vi "Relay_Checker.vi"(0 "TSM context":T1) -> (15 "error out":errorcluster)   [LabVIEW 2019]
uses:
  <vilib>/NI_TestStand_SemiconductorModule/NI_TestStand_Semiconductor_Module.lvlibp/PinMap/General/SemiconductorModuleContext.ctl
  Common/Instrument Control/DCPower/TSM/TSM SSC DCPower.ctl
  <vilib>/NI_TestStand_SemiconductorModule/NI_TestStand_Semiconductor_Module.lvlibp/PinMap/PinQueryContext/MultiplePinMultipleSessionQueryContext/MultiplePinMultipleSessionQueryContext.lvclass
  Common/Instrument Control/DCPower/SSC DCPower/SSC DCPower.ctl
  Common/Instrument Control/Shared SubVIs/TSM Pin Abstraction/TSM Pin Information.ctl
  Common/Instrument Control/Shared SubVIs/TSM Pin Abstraction/TSM Pin Type Identifier.ctl
  Common/Instrument Control/Shared SubVIs/TSM Pin Abstraction/TSM Expanded Pin Information.ctl
  Common/Instrument Control/Relay/Pin Map/TSM Relay.ctl
  <vilib>/NI_TestStand_SemiconductorModule/NI_TestStand_Semiconductor_Module.lvlibp/1abvi3w/instr.lib/niSwitch/niswitch.llb/niSwitch Relay Action.ctl
  Common/Instrument Control/Relay/Pin Map/TSM Relay PinTypeInfo.vi
  <vilib>/NI_TestStand_SemiconductorModule/NI_TestStand_Semiconductor_Module.lvlibp/PinMap/Advanced/GetRelaysInRelayGroup(s).vi
  <vilib>/NI_TestStand_SemiconductorModule/NI_TestStand_Semiconductor_Module.lvlibp/PinMap/Advanced/GetRelaysInRelayGroups.vi
  <vilib>/Utility/High Resolution Polling Wait.vi
  Common/Instrument Control/DCPower/SSC DCPower/Control/SSC DCPower Abort.vi
  Common/Instrument Control/DCPower/SSC DCPower/Source/SSC DCPower Configure Output Connected.vi
  Common/Instrument Control/DCPower/SSC DCPower/Source/SSC DCPower Configure Output Enabled.vi
  Common/Instrument Control/DCPower/SSC DCPower/Control/SSC DCPower Initiate.vi
  <vilib>/NI_TestStand_SemiconductorModule/NI_TestStand_Semiconductor_Module.lvlibp/PinMap/Relay Driver/ControlRelay(s).vi
  <vilib>/NI_TestStand_SemiconductorModule/NI_TestStand_Semiconductor_Module.lvlibp/PinMap/Relay Driver/ControlRelaysSingleAction.vi
  <vilib>/NI_TestStand_SemiconductorModule/NI_TestStand_Semiconductor_Module.lvlibp/PinMap/General/Publish/PublishDataDoubleFunctionalTest.vi
  TSM Context Data Access/TSM Context Data Access.lvclass
  <vilib>/NI_TestStand_SemiconductorModule/NI_TestStand_Semiconductor_Module.lvlibp
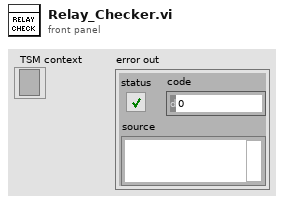
[diagram p1: front panel]
types:
  T1 = typedef "NI_TestStand_Semiconductor_Module.lvlibp/SemiconductorModuleContext.ctl" = refnum<k7>
  T2 = cluster{"unloaded12VRLY":dbl[], "vdiode":dbl[], "RelayDrop":dbl[][]}
  T3 = typedef "TSM SSC DCPower.ctl" = cluster{"Pin Query Context":refnum<class "MultiplePinMultipleSessionQueryContext.lvclass">, "SSC":T4[], "Site Numbers":i32[], "Pins":T5[], "Pins Expanded":T7[]}
  T4 = typedef "SSC DCPower.ctl" = cluster{"Session":refnum<k15>, "Chan":string, "Channel List":string}
  T5 = typedef "TSM Pin Information.ctl" = cluster{"Pin":tag, "Type":T6, "Count":i32}
  T6 = typedef "TSM Pin Type Identifier.ctl" = enum8{"DUT Pin", "System Pin", "Pin Group", "Not Determined"}
  T7 = typedef "TSM Expanded Pin Information.ctl" = cluster{"Pin":tag, "Type":T6, "Index":i32}
  T8 = typedef "TSM Relay.ctl" = cluster{"TSM Context":T1, "Relays":tag[]}
  T9 = cluster{"RLY12V_MEAS":T3, "Relays Filtered Pins":string[], "Relay Pin Sessions":T8[]}
  T10 = typedef "NI_TestStand_Semiconductor_Module.lvlibp/niSwitch Relay Action.ctl" = i32
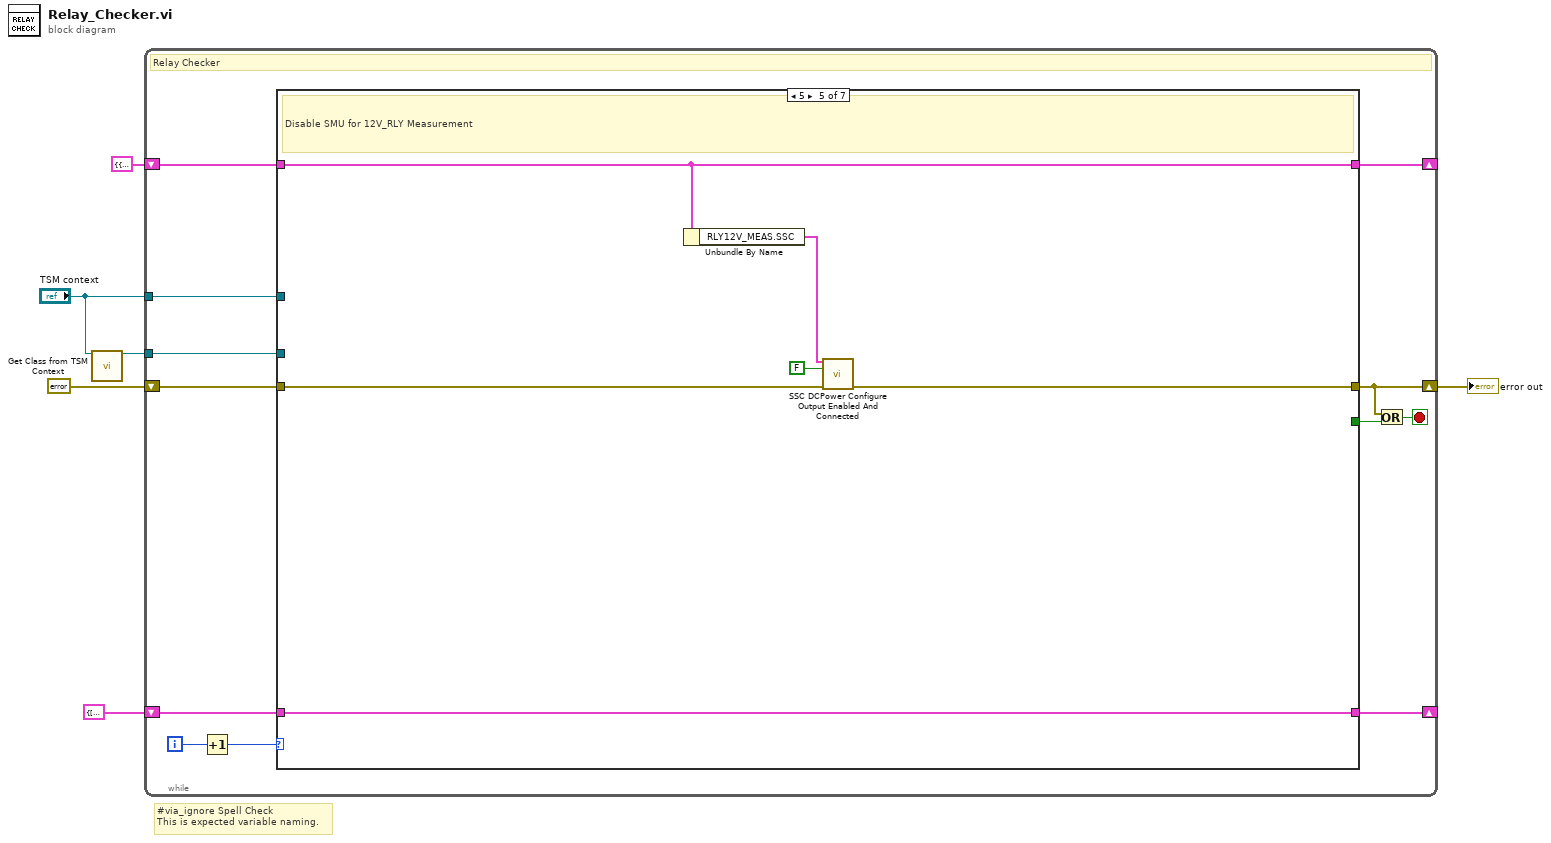
[diagram p0: block diagram]
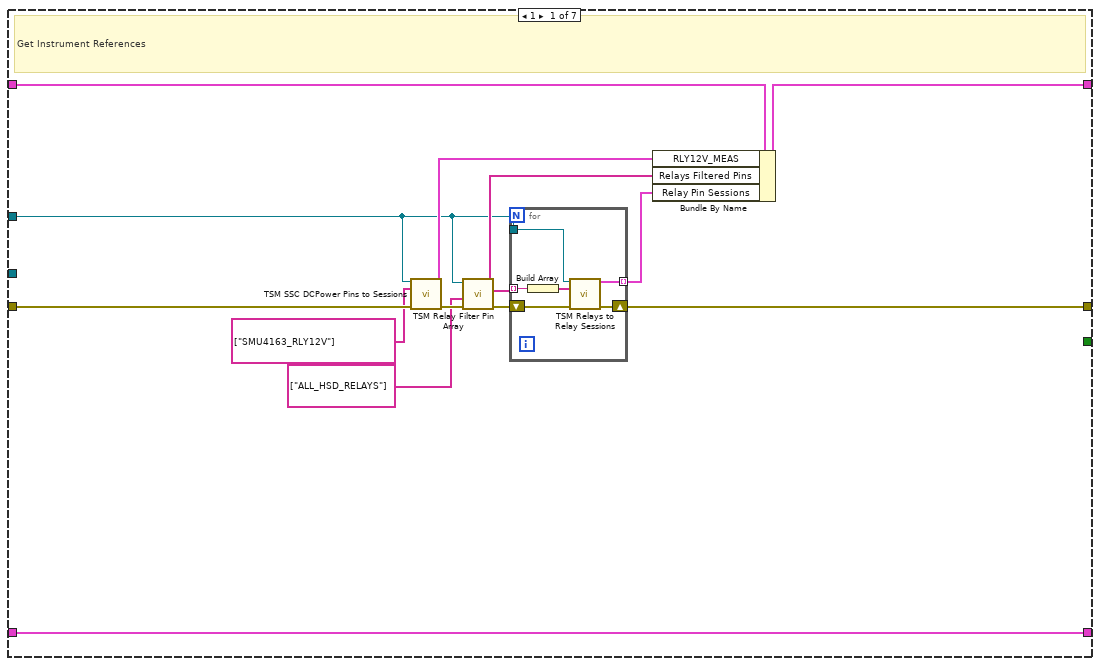
[diagram p2: hidden frame]
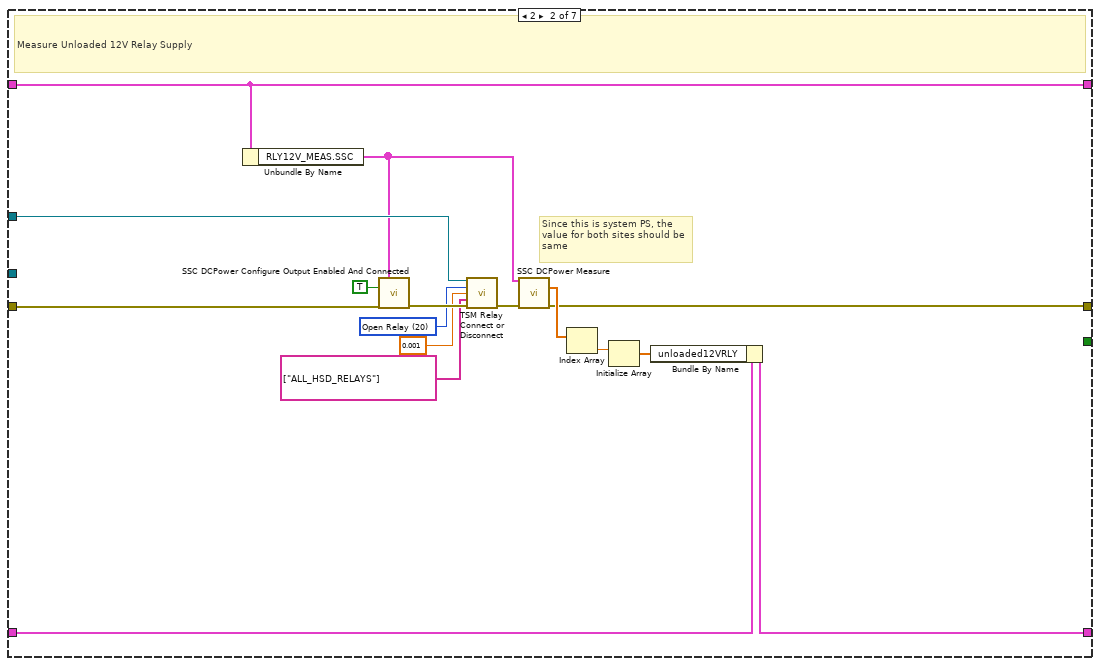
[diagram p3: hidden frame]
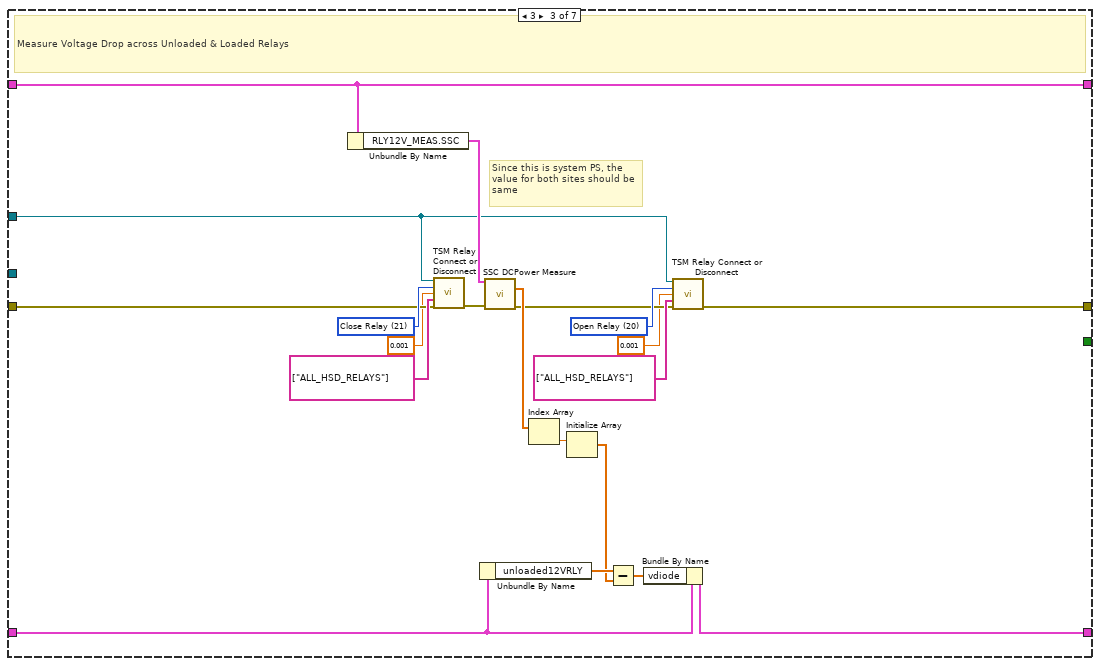
[diagram p4: hidden frame]
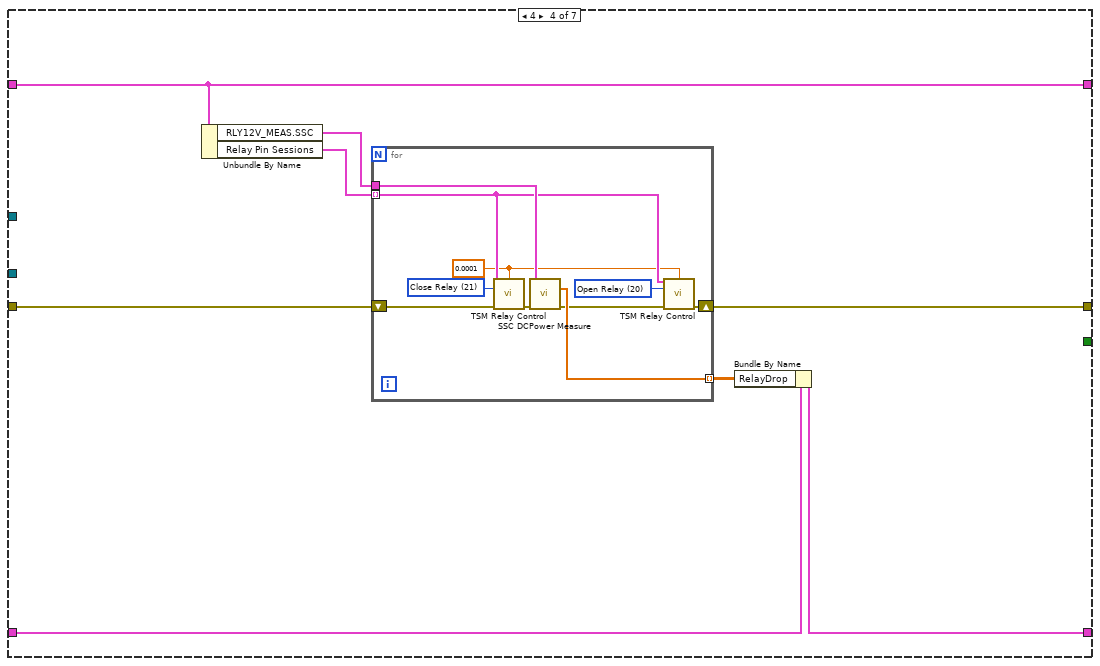
[diagram p5: hidden frame]
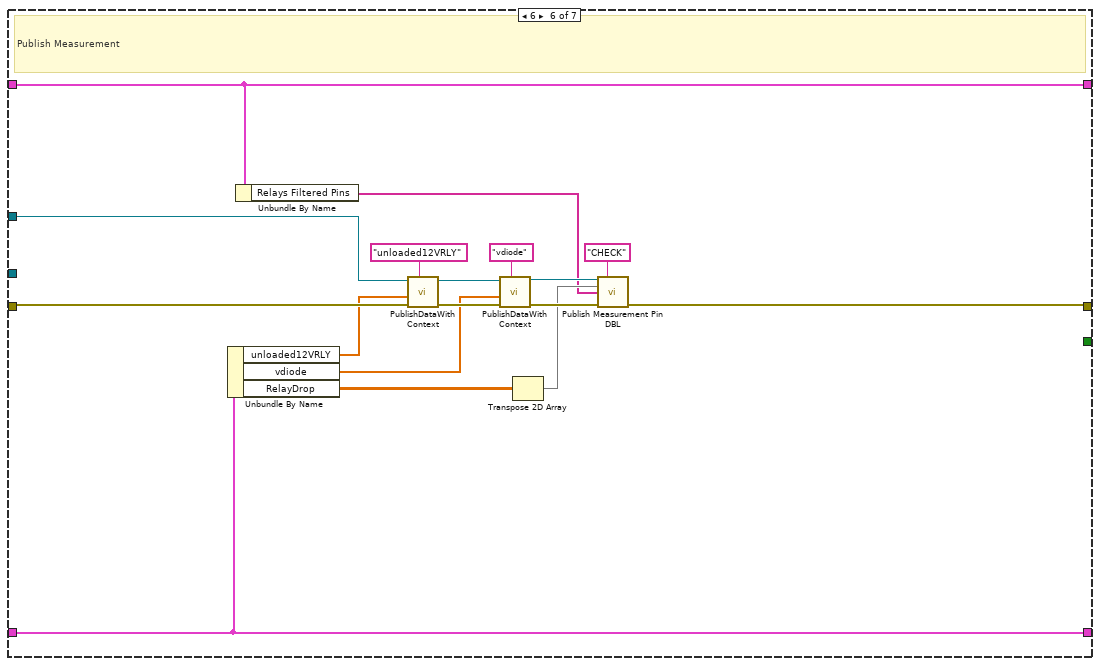
[diagram p6: hidden frame]
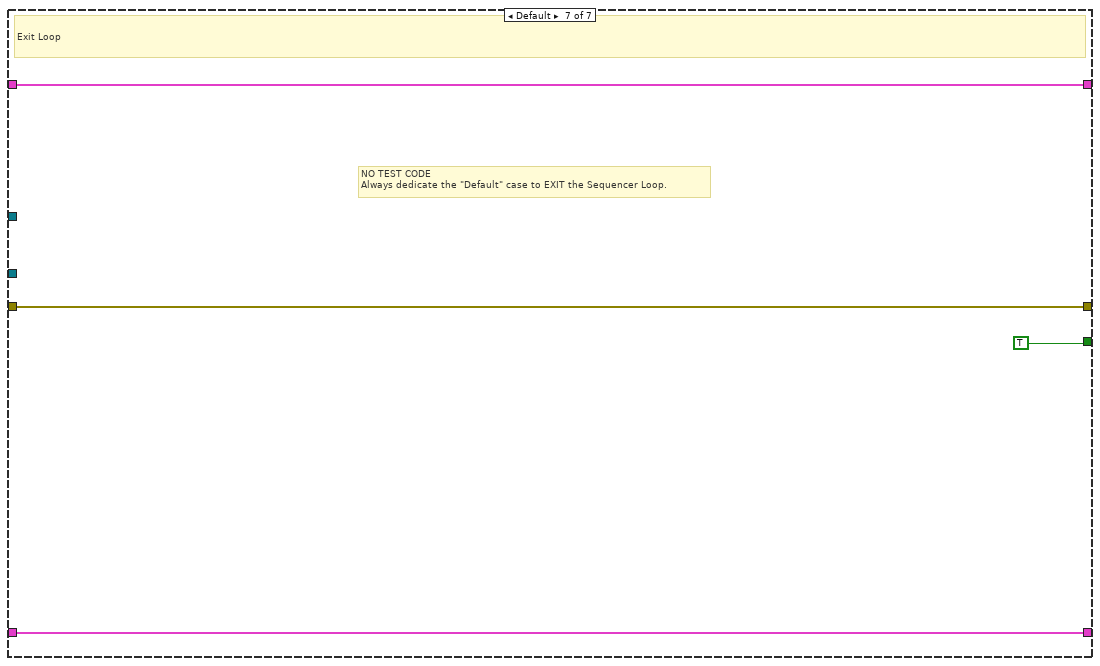
[diagram p7: hidden frame]
diagram:
  # "#via_ignore Spell Check\nThis is expected variable naming."
  n1 = call "Get Class from TSM Context.vi"("TSM Context"="TSM context") -> ("Global Memory Class"=w2:refnum<class "TSM Context Data Access.lvclass">)  [unwired: 14 in]
  n2 = while {
    shift-right: [w10] -> w6
    shift-left: errorcluster {"status"=FALSE, "code"=0, "source"=""} ("error in") -> [w17]
    tunnel: "TSM context" -> [w15]
    shift-right: [w12] -> _
    shift-left: T9 {"RLY12V_MEAS"={"Pin Query Context"=refnum, "SSC"=[], "Site Numbers"=[], "Pins"=[], "Pins Expanded"=[]}, "Relays Filtered Pins"=[], "Relay Pin Sessions"=[]} -> [w13]
    shift-right: [w9] -> _
    shift-left: T2 {"unloaded12VRLY"=[], "vdiode"=[], "RelayDrop"=[]} -> [w8]
    tunnel: w2 -> [w7]
    i -> [w18]
    stop <- w11 stop-if-true
    # "Relay Checker"
    n3 = Increment(x=w18) -> (x+1=w16:i32)
    n4 = case shown="5" w16 {
      tunnel: [w22 w42 w58 w77 w92 w100 w117] -> w10
      tunnel: w17 -> [w31 w41 w68 w79 w93 w110 w117]
      tunnel: w15 -> [w20 w48 w57 _ _ w109 _]
      tunnel: [_ _ _ _ _ _ TRUE] -> w14
      tunnel: w13 -> [w30 w51 w67 w81 w95 w104 w116]
      tunnel: [w29 w51 w67 w81 w95 w104 w116] -> w12
      tunnel: [w21 w43 w62 w74 w97 w108 w115] -> w9
      tunnel: w8 -> [w21 w45 w54 w76 w97 w108 w115]
      tunnel: w7 -> [_ _ _ _ _ _ _]
      frame 1 {
        # "Get Instrument References"
        n5 = call "TSM SSC DCPower Pins to Sessions.vi"("TSM context"=w20, "Pins"=tag[] ["SMU4163_RLY12V"], "error in"=w31) -> ("DCPower TSM Out"=w28:T3, "error out"=w26:errorcluster)  [unwired: 11 in]
        n6 = call "TSM Relay Filter Pin Array.vi"("error in"=w26, "Pins"=string[] ["ALL_HSD_RELAYS"], "TSM context in"=w20) -> ("error out"=w25:errorcluster, "Filtered Pins Array"=w24:string[])  [unwired: 4 in, 3 out]
        n7 = for {
          shift-right: [w34] -> w22
          shift-left: w25 -> [w37]
          tunnel: w24 -> [w36] mode=indexing
          tunnel: [w35] -> w23 mode=indexing
          tunnel: w20 -> [w32]
          n8 = Build Array(w36) -> (w33:string[])
          n9 = call "TSM Relays to Relay Sessions.vi"("TSM Context"=w32, "Relays"=w33, "error in (no error)"=w37) -> ("TSM Relay Out"=w35:T8, "error out"=w34:errorcluster)  [unwired: 11 in]
        }
        n10 = Bundle By Name(cluster=w30, "RLY12V_MEAS"=w28, "Relays Filtered Pins"=w24, "Relay Pin Sessions"=w23) -> (w29:T9)
      }
      frame 2 {
        w49 = T10 20 items=["Open Relay"=20, "Close Relay"=21] ("Relay Action")
        # "Since this is system PS, the value for both sites should be same"
        # "Measure Unloaded 12V Relay Supply"
        n11 = Unbundle By Name(w51) -> ("RLY12V_MEAS.SSC"=w38:T4[])
        n12 = call "SSC DCPower Configure Output Enabled And Connected.vi"("DCPower SSC in"=w38, "Output Enabled And Connected"=TRUE, "error in"=w41) -> ("error out"=w52:errorcluster)  [unwired: 11 in, 1 out]
        n13 = call "TSM Relay Connect or Disconnect.vi"("TSM context"=w48, "Relay Action"=w49, "Settling Time (s)"=0.001 ("seconds to wait"), "Relays"=tag[] ["ALL_HSD_RELAYS"], "error in"=w52) -> ("error out"=w39:errorcluster)  [unwired: 9 in, 1 out]
        n14 = call "SSC DCPower Measure.vi"("DCPower SSC in"=w38, "error in"=w39) -> ("Voltage Measurements (V)"=w47:dbl[], "error out"=w42:errorcluster)  [unwired: 10 in, 2 out]
        n15 = Index Array(array=w47) -> (element=w46:dbl)  [unwired: 1 in]
        n16 = Initialize Array(w46) -> (w44:dbl[])  [unwired: 1 in]
        n17 = Bundle By Name(cluster=w45, "unloaded12VRLY"=w44) -> (w43:T2)
      }
      frame 3 {
        w60 = T10 20 items=["Open Relay"=20, "Close Relay"=21] ("Relay Action")
        w72 = T10 21 items=["Open Relay"=20, "Close Relay"=21] ("Relay Action")
        # "Since this is system PS, the value for both sites should be same"
        # "Measure Voltage Drop across Unloaded & Loaded Relays"
        n18 = Unbundle By Name(w67) -> ("RLY12V_MEAS.SSC"=w66:T4[])
        n19 = call "TSM Relay Connect or Disconnect.vi"("TSM context"=w57, "Relay Action"=w72, "Settling Time (s)"=0.001, "Relays"=tag[] ["ALL_HSD_RELAYS"], "error in"=w68) -> ("error out"=w71:errorcluster)  [unwired: 9 in, 1 out]
        n20 = Unbundle By Name(w54) -> ("unloaded12VRLY"=w64:dbl[])
        n21 = call "SSC DCPower Measure.vi"("DCPower SSC in"=w66, "error in"=w71) -> ("Voltage Measurements (V)"=w70:dbl[], "error out"=w59:errorcluster)  [unwired: 10 in, 2 out]
        n22 = Index Array(array=w70) -> (element=w69:dbl)  [unwired: 1 in]
        n23 = Initialize Array(w69) -> (w63:dbl[])  [unwired: 1 in]
        n24 = Subtract(x=w64, y=w63) -> (x-y=w65:dbl[])
        n25 = Bundle By Name(cluster=w54, "vdiode"=w65) -> (w62:T2)
        n26 = call "TSM Relay Connect or Disconnect.vi"("TSM context"=w57, "Relay Action"=w60, "Settling Time (s)"=0.001, "Relays"=tag[] ["ALL_HSD_RELAYS"], "error in"=w59) -> ("error out"=w58:errorcluster)  [unwired: 9 in, 1 out]
      }
      frame 4 {
        n27 = Unbundle By Name(w81) -> ("RLY12V_MEAS.SSC"=w80:T4[], "Relay Pin Sessions"=w78:T8[])
        n28 = for {
          tunnel: w80 -> [w91]
          shift-right: [w83] -> w77
          shift-left: w79 -> [w89]
          tunnel: [w90] -> w75 mode=indexing
          tunnel: w78 -> [w85] mode=indexing
          w84 = T10 20 items=["Open Relay"=20, "Close Relay"=21] ("Relay Action")
          w82 = 0.0001 ("Settling Time (s)")
          w88 = T10 21 items=["Open Relay"=20, "Close Relay"=21] ("Relay Action")
          n29 = call "TSM Relay Control.vi"("Relay TSM in"=w85, "Settling Time (s)"=w82, "Relay Action"=w88, "error in"=w89) -> ("error out"=w87:errorcluster)  [unwired: 11 in]
          n30 = call "SSC DCPower Measure.vi"("DCPower SSC in"=w91, "error in"=w87) -> ("Voltage Measurements (V)"=w90:dbl[], "error out"=w86:errorcluster)  [unwired: 10 in, 2 out]
          n31 = call "TSM Relay Control.vi"("Relay TSM in"=w85, "Settling Time (s)"=w82, "Relay Action"=w84, "error in"=w86) -> ("error out"=w83:errorcluster)  [unwired: 11 in]
        }
        n32 = Bundle By Name(cluster=w76, "RelayDrop"=w75) -> (w74:T2)
      }
      frame 5 {
        # "Disable SMU for 12V_RLY Measurement"
        n33 = Unbundle By Name(w95) -> ("RLY12V_MEAS.SSC"=w94:T4[])
        n34 = call "SSC DCPower Configure Output Enabled And Connected.vi"("DCPower SSC in"=w94, "Output Enabled And Connected"=FALSE, "error in"=w93) -> ("error out"=w92:errorcluster)  [unwired: 11 in, 1 out]
      }
      frame 6 {
        # "Publish Measurement"
        n35 = Unbundle By Name(w108) -> ("unloaded12VRLY"=w107:dbl[], "vdiode"=w106:dbl[], "RelayDrop"=w102:dbl[][])
        n36 = Unbundle By Name(w104) -> ("Relays Filtered Pins"=w98:string[])
        n37 = call-poly <vilib>:"PublishDataWithContext.vi"("Published Data Id"="unloaded12VRLY", "error in (no error)"=w110, "Data In"=w107, "Semiconductor Module Context"=w109) -> ("error out"=w112:errorcluster, "Semiconductor Module Context Out"=w113:T1)  [unwired: 6 in]
        n38 = call-poly <vilib>:"PublishDataWithContext.vi"("Published Data Id"="vdiode", "error in (no error)"=w112, "Data In"=w106, "Semiconductor Module Context"=w113) -> ("error out"=w105:errorcluster, "Semiconductor Module Context Out"=w103:T1)  [unwired: 6 in]
        n39 = Transpose 2D Array(2D array=w102) -> (transposed array=w101:dbl[][])
        n40 = call "Publish Measurement Pin DBL.vi"("TSM context in"=w103, "Published Data Id In"="CHECK", "Measurement Data (row - per site)"=w101, "Expanded Pin List in"=w98, "error in"=w105) -> ("error out"=w100:errorcluster)  [unwired: 7 in, 3 out]
      }
      frame Default {
        # "NO TEST CODE\nAlways dedicate the \"Default\" case to EXIT the Sequencer Loop."
        # "Exit Loop"
      }
    }
    n41 = Or(x=w10, y=w14) -> (x .or. y?=w11:bool)
  }
  "error out" <- w6
